vi "APC_9056_O2Control.vi"(1 "LoadIni?":bool, 2 "PC_ControlSettings":T1={"Spark advance [CADBTDC]"=0.0, "Pref"=0.0, "O2ref"=0.0, "DI advance [CADBTDC]"=0.0, "DI duration [ms] "=0.0, "CO2ref"=0.0, "PFI duration [ms]"=0.0, "IMEP ref"=0.0, "Speed ref"=0.0, "IGN enable"=TRUE, "DI enable"=TRUE, "CL PFI\n lambda"=TRUE, "CL PFI\nIMEP"=FALSE, "Activate\ncylinder"=[FALSE, FALSE, FALSE, FALSE, FALSE, FALSE], "Force idling"=FALSE, "Force motoring"=FALSE, "ETP resync"=FALSE, "Requested mode"=0, "Clear Sync Errors"=FALSE, "toggle TDC"=FALSE, "l ref"=0.0, "PID control references"={"NG"=FALSE, "Ar"=FALSE, "O2"=FALSE, "Intake vent"=FALSE, "Cross vent"=FALSE, "Exhaust vent"=FALSE, "NG control mode"=0, "NG-FC-001-REF"=0.0, "WF-OA-002-REF"=0.0, "IMEP-REF"=0.0, "Nm-REF"=0.0, "Ar control mode"=0, "AR-PC-002-REF"=0.0, "WF-PT-004-REF"=0.0, "O2 control mode"=0, "O2-FC-001-REF"=0.0, "WF-OA-001-REF"=0.0, "Tcoolant control  mode"=0, "EC-FC-001-REF"=0.0, "EC-TT-001-REF"=0.0, "Texh control mode"=0, "SW-FC-004-REF"=0.0, "SW-FT-002-REF"=0.0, "WF-TT-004-REF"=0.0, "Toil control mode"=0, "SW-FC-009-REF"=0.0, "SW-FT-004-REF"=0.0, "EO-TT-001-REF"=0.0, "AIC201_CO2_ConcTarget"=0.0, "O2_FF_NG"=FALSE, "Dyno control mode"=0, "Membrane control mode"=0, "AR-FT-001-REF"=0.0, "MTR modbus floats"=[0.0, 0.0, 0.0, 0.0, 0.0, 0.0, 0.0, 0.0, 0.0, 0.0, 0.0, 0.0, 0.0, 0.0, 0.0, 0.0, 0.0, 0.0, 0.0], "MTR modbus u16"=[0, 0, 0, 0, 0, 0, 0], "MTR HB"=FALSE, "PC_HB"=FALSE, "EMERGENCY STOP"=FALSE}, "CA50setpoint [CADATDC]"=0.0, "CA50 control"=TRUE, "Knock control"=TRUE, "CLEAR EMERGENCY STOP"=FALSE, "EMERGENCY STOP"=FALSE}, 3 "input cluster":T3) -> (0 "O2-FC-001-REF":dbl format="%.2f")   [LabVIEW 2020]
uses:
  controls/APC_PIDCluster.ctl
  controls/APC_ControlSettings.ctl
  controls/APC_PIDcontrolSettings.ctl
  controls/APC_cascadePIDsettings.ctl
  <vilib>/addons/control/pid/pid.llb/PID Advanced (DBL).vi
  <vilib>/Utility/xml.llb/Read From XML File(string).vi
  <vilib>/Utility/xml.llb/Write to XML File(string).vi
  <vilib>/addons/control/pid/NI_PID_pid.lvlib
panel:
  out "direct?":bool
  out "Direct control":dbl format="%.2f"
  in  "O2-FC-001-REF (manual)":dbl
  in  "O2/NG":dbl=3.0
  in  "compensate NG":bool
  in  "FT/FC?":bool
  in  "save":bool
  in  "load":bool
  out "O2 control mode":u8
  out "EC-TT-001":dbl
  in  "FF control":dbl format="%.2f"
  in  "reinitialize? (F)":bool
  in  "WF-OA-001-O2corr-REF (manual)":dbl
  in  "O2 control mode (manual)":u8
  in  "PID gains":T4={"proportional gain (Kc)"=1.0, "integral time (Ti, min)"=0.01, "derivative time (Td, min)"=0.0} {"derivative time (Td, min)" format="%.3f"; "integral time (Ti, min)" format="%.3f"; "proportional gain (Kc)" format="%.3f"}
  in  "PID setpoint range":cluster{"setpoint high":dbl, "setpoint low":dbl}={"setpoint high"=100.0, "setpoint low"=0.0} {"setpoint high" format="%.2f"; "setpoint low" format="%.2f"}
  in  "PID output range":cluster{"output high":dbl, "output low":dbl}={"output high"=100.0, "output low"=-100.0} {"output low" format="%.2f"; "output high" format="%.2f"}
  in  "Override PC PID references":bool
  in  "Safe mode control":dbl format="%.2f"
  in  "learn?":bool
  out "CL on?":bool
  out "setpoint":dbl format="%.2f"
  # "O2 control"
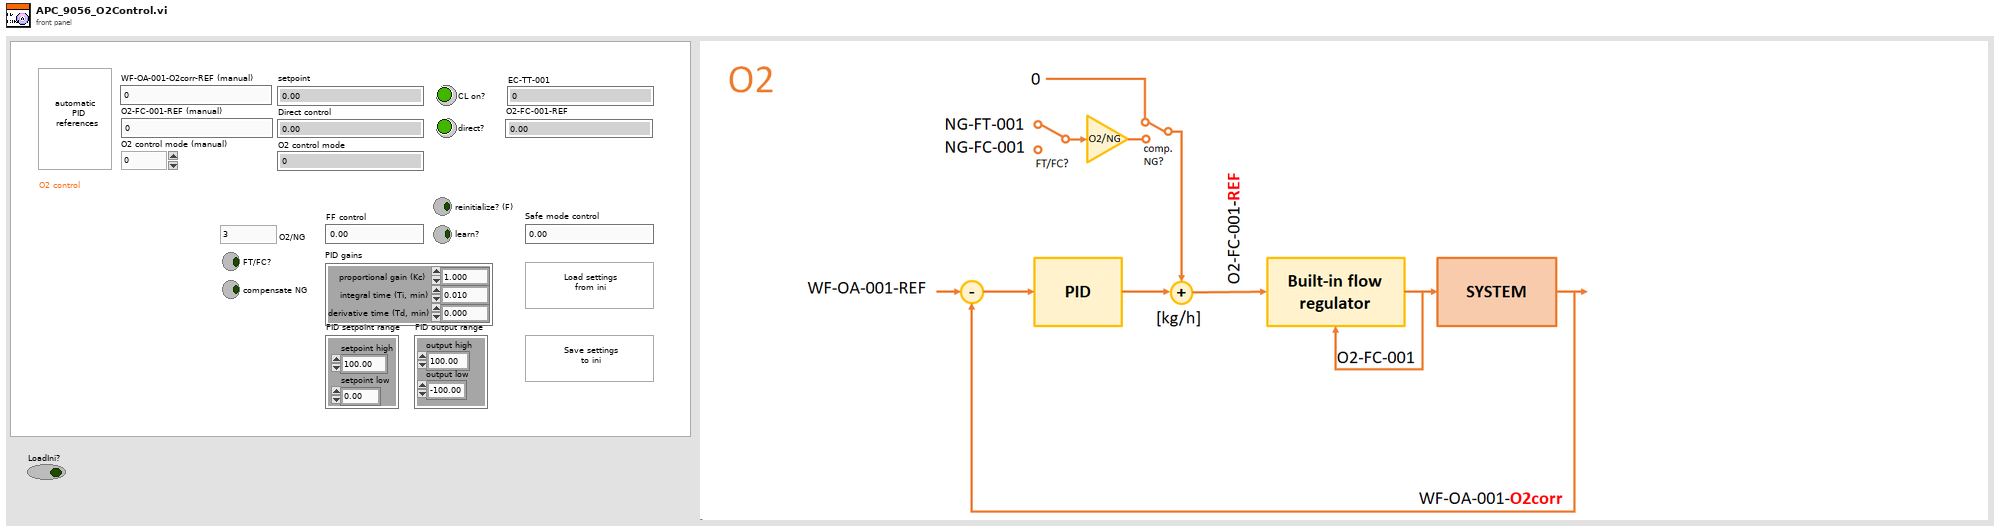
[diagram p1: front panel]
types:
  T1 = typedef "APC_ControlSettings.ctl" = cluster{"Spark advance [CADBTDC]":dbl, "Pref":dbl, "O2ref":dbl, "DI advance [CADBTDC]":dbl, "DI duration [ms] ":dbl, "CO2ref":dbl, "PFI duration [ms]":dbl, "IMEP ref":dbl, "Speed ref":dbl, "IGN enable":bool, "DI enable":bool, "CL PFI\n lambda":bool, "CL PFI\nIMEP":bool, "Activate\ncylinder":bool[], "Force idling":bool, "Force motoring":bool, "ETP resync":bool, "Requested mode":i8, "Clear Sync Errors":bool, "toggle TDC":bool, "l ref":dbl, "PID control references":T2, "CA50setpoint [CADATDC]":dbl, "CA50 control":bool, "Knock control":bool, "CLEAR EMERGENCY STOP":bool, "EMERGENCY STOP":bool}
  T2 = typedef "APC_PIDcontrolSettings.ctl" = cluster{"NG":bool, "Ar":bool, "O2":bool, "Intake vent":bool, "Cross vent":bool, "Exhaust vent":bool, "NG control mode":u8, "NG-FC-001-REF":dbl, "WF-OA-002-REF":dbl, "IMEP-REF":dbl, "Nm-REF":dbl, "Ar control mode":u8, "AR-PC-002-REF":dbl, "WF-PT-004-REF":dbl, "O2 control mode":u8, "O2-FC-001-REF":dbl, "WF-OA-001-REF":dbl, "Tcoolant control  mode":u8, "EC-FC-001-REF":dbl, "EC-TT-001-REF":dbl, "Texh control mode":u8, "SW-FC-004-REF":dbl, "SW-FT-002-REF":dbl, "WF-TT-004-REF":dbl, "Toil control mode":u8, "SW-FC-009-REF":dbl, "SW-FT-004-REF":dbl, "EO-TT-001-REF":dbl, "AIC201_CO2_ConcTarget":dbl, "O2_FF_NG":bool, "Dyno control mode":u8, "Membrane control mode":u8, "AR-FT-001-REF":dbl, "MTR modbus floats":sgl[], "MTR modbus u16":u16[], "MTR HB":bool, "PC_HB":bool, "EMERGENCY STOP":bool}
  T3 = typedef "APC_PIDCluster.ctl" = cluster{"AR-FT-001":dbl, "O2-FC-001":dbl, "SW-FT-004":dbl, "SW-FT-002":dbl, "WF-OA-002":dbl, "WF-PT-004":dbl, "WF-OA-001":dbl, "EC-TT-001":dbl, "WF-TT-004":dbl, "EC-FC-001":dbl, "NG-FC-001":dbl, "EO-TT-001":dbl, "SW-FC-008":dbl, "SW-FC-004":dbl, "IMEPn6":dbl, "TORQUE":dbl, "CylPresWarnings":dbl, "CylPresErrors":dbl, "NG-FT-001":dbl, "EngineSpeed_rpm":dbl}
  T4 = cluster{"proportional gain (Kc)":dbl, "integral time (Ti, min)":dbl, "derivative time (Td, min)":dbl}
  T5 = typedef "APC_cascadePIDsettings.ctl" = cluster{"HL FF control":dbl, "LL FF control":dbl, "HL PID gains":cluster{"proportional gain (Kc)":dbl, "integral time (Ti, min)":dbl, "derivative time (Td, min)":dbl}, "LL PID gains":cluster{"proportional gain (Kc)":dbl, "integral time (Ti, min)":dbl, "derivative time (Td, min)":dbl}, "HL PID setpoint range":cluster{"setpoint high":dbl, "setpoint low":dbl}, "HL PID output range":cluster{"output high":dbl, "output low":dbl}, "LL PID setpoint range":cluster{"setpoint high":dbl, "setpoint low":dbl}, "LL PID output range":cluster{"output high":dbl, "output low":dbl}, "Safe mode control":dbl}
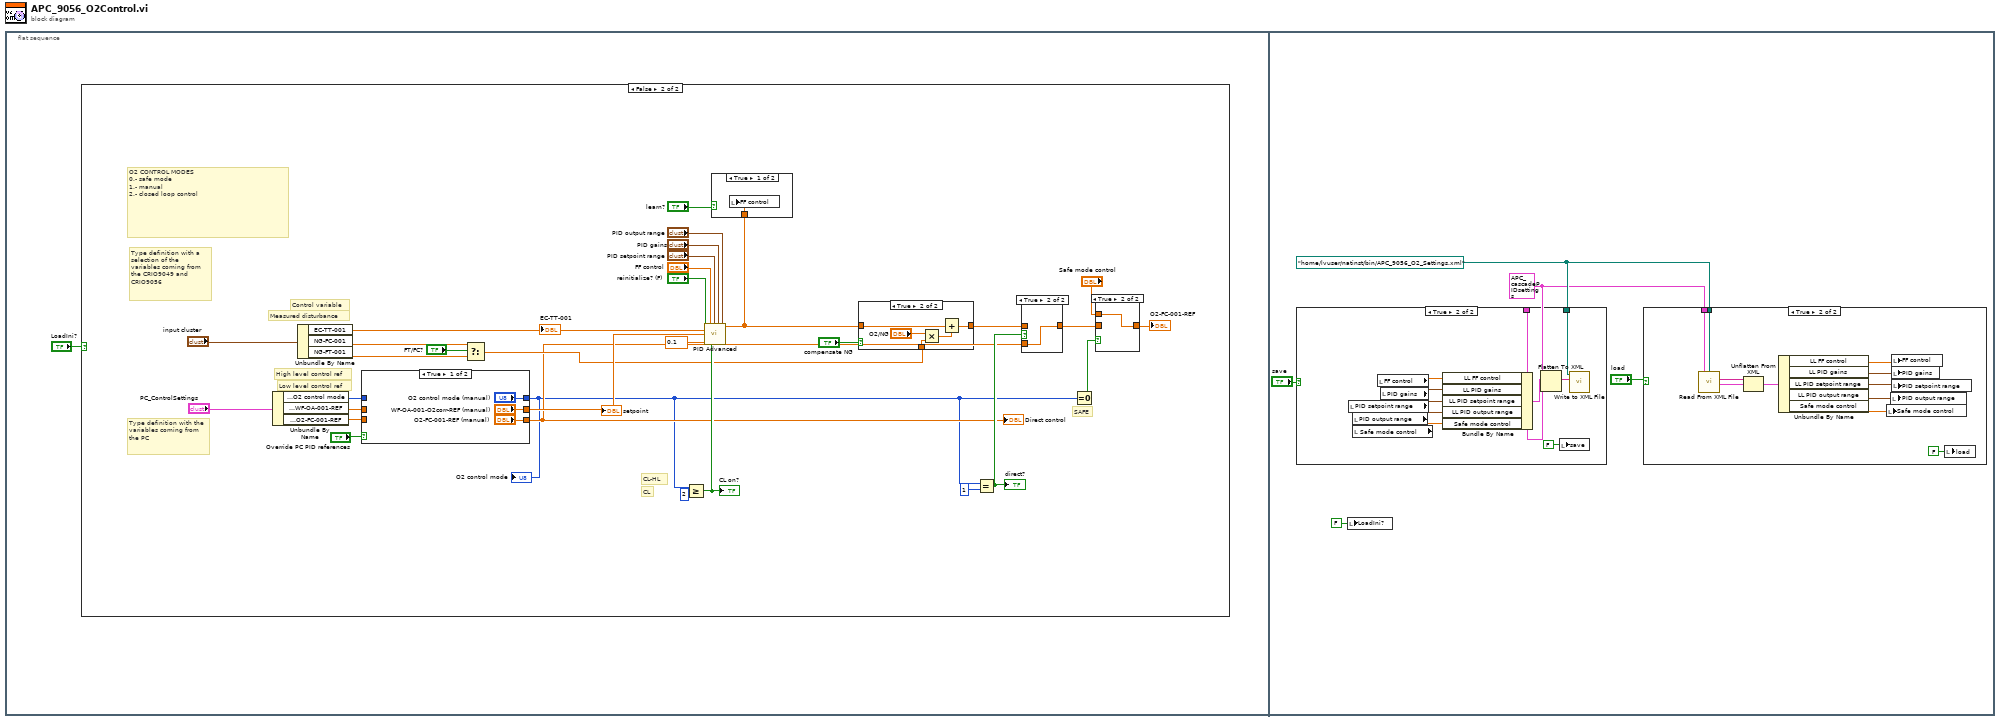
[diagram p0: block diagram]
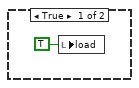
[diagram p2: hidden frame]
diagram:
  n1 = flat-sequence {
    frame #0 {
      n2 = case shown="False" "LoadIni?" {
        frame True {
          n3 = local write "load"(TRUE ("load")) -> ()
        }
        frame False {
          # "Type definition with a selection of the variables coming from the CRIO9049 and CRIO9056"
          # "Type definition with the variables coming from the PC"
          # "Low level control ref"
          # "Measured disturbance"
          # "High level control ref"
          # "Control variable"
          # "SAFE"
          # "CL-HL"
          # "CL"
          # "O2 CONTROL MODES\n0.- safe mode\n1.- manual\n2.- closed loop control"
          n4 = Unbundle By Name("PC_ControlSettings") -> ("PID control references.O2 control mode"=w22:u8, "PID control references.WF-OA-001-REF"=w21:dbl, "PID control references.O2-FC-001-REF"=w9:dbl)
          n5 = Unbundle By Name("input cluster") -> ("EC-TT-001"=w19:dbl, "NG-FC-001"=w15:dbl, "NG-FT-001"=w14:dbl)
          "EC-TT-001" <- w19
          n6 = case shown="True" "Override PC PID references" {
            tunnel: w22 -> [_ w51]
            tunnel: w21 -> [_ w50]
            tunnel: ["O2 control mode (manual)" w51] -> w3
            tunnel: ["WF-OA-001-O2corr-REF (manual)" w50] -> w16
            tunnel: w9 -> [_ w49]
            tunnel: ["O2-FC-001-REF (manual)" w49] -> w4
            frame True {
            }
            frame False {
            }
          }
          "setpoint" <- w16
          "O2 control mode" <- w3
          "Direct control" <- w4
          n7 = Select(t=w15, s="FT/FC?", f=w14) -> (s? t:f=w10:dbl)
          n8 = Greater Or Equal?(x=w3, y=u8 2) -> (x >= y?=w32:bool)
          "CL on?" <- w32
          n9 = call-poly <vilib>:"PID Advanced.vi"("setpoint"=w16, "output range"="PID output range", "auto? (T)"=w32, "manual control"="FF control", "process variable"=w19, "setpoint range"="PID setpoint range", "PID gains"="PID gains", "dt (s)"=0.1, "reinitialize? (F)"="reinitialize? (F)") -> ("output"=w11:dbl)  [unwired: 5 in, 1 out]
          n10 = case shown="True" "learn?" {
            tunnel: w11 -> [w43 _]
            frame True {
              n11 = local write "FF control"(w43) -> ()
            }
            frame False {
            }
          }
          n12 = case shown="True" "compensate NG" {
            tunnel: w11 -> [w37 w41]
            tunnel: [w37 w42] -> w5
            tunnel: w10 -> [_ w39]
            frame False {
            }
            frame True {
              n13 = Multiply(x="O2/NG", y=w39) -> (x*y=w40:dbl)
              n14 = Add(x=w41, y=w40) -> (x+y=w42:dbl)
            }
          }
          n15 = Equal?(x=w3, y=u8 1) -> (x = y?=w7:bool)
          "direct?" <- w7
          n16 = case shown="True" w7 {
            tunnel: [w35 w36] -> w6
            tunnel: w5 -> [w35 _]
            tunnel: w4 -> [_ w36]
            frame False {
            }
            frame True {
            }
          }
          n17 = Equal To 0?(x=w3) -> (x = 0?=w34:bool)
          n18 = case shown="True" w34 {
            tunnel: [w44 w45] -> w28
            tunnel: "Safe mode control" -> [_ w45]
            tunnel: w6 -> [w44 _]
            frame False {
            }
            frame True {
            }
          }
          "O2-FC-001-REF" <- w28
        }
      }
    }
    frame #1 {
      w54 = path "/home/lvuser/natinst/bin/APC_9056_O2_Settings.xml" ("XML File Path")
      w53 = T5 {"HL FF control"=0.0, "LL FF control"=0.0, "HL PID gains"={"proportional gain (Kc)"=1.0, "integral time (Ti, min)"=0.01, "derivative time (Td, min)"=0.0}, "LL PID gains"={"proportional gain (Kc)"=1.0, "integral time (Ti, min)"=0.01, "derivative time (Td, min)"=0.0}, "HL PID setpoint range"={"setpoint high"=100.0, "setpoint low"=0.0}, "HL PID output range"={"output high"=0.0, "output low"=0.0}, "LL PID setpoint range"={"setpoint high"=100.0, "setpoint low"=0.0}, "LL PID output range"={"output high"=10.0, "output low"=-10.0}, "Safe mode control"=0.0} ("Cluster")
      n19 = case shown="True" "save" {
        tunnel: w54 -> [_ w69]
        tunnel: w53 -> [_ w68]
        frame False {
        }
        frame True {
          n20 = local read "PID setpoint range"() -> (w74:cluster{"setpoint high":dbl, "setpoint low":dbl})
          n21 = local read "PID output range"() -> (w73:cluster{"output high":dbl, "output low":dbl})
          n22 = local read "Safe mode control"() -> (w72:dbl)
          n23 = local read "FF control"() -> (w76:dbl)
          n24 = local read "PID gains"() -> (w75:T4)
          n25 = Bundle By Name(cluster=w68, "LL FF control"=w76, "LL PID gains"=w75, "LL PID setpoint range"=w74, "LL PID output range"=w73, "Safe mode control"=w72) -> (w71:T5)
          n26 = Flatten To XML(6:w71) -> (2:w70:string)
          n27 = local write "save"(FALSE ("load")) -> ()
          n28 = call-poly <vilib>:"Write to XML File.vi"("XML Input"=w70, "XML File Path"=w69) -> ()  [unwired: 7 in, 3 out]
        }
      }
      n29 = local write "LoadIni?"(FALSE ("LoadIni?")) -> ()
      n30 = case shown="True" "load" {
        tunnel: w54 -> [_ w65]
        tunnel: w53 -> [_ w64]
        frame False {
        }
        frame True {
          n31 = call-poly <vilib>:"Read From XML File.vi"("XML File Path"=w65) -> ("XML Elements"=w66:string)  [unwired: 8 in, 2 out]
          n32 = Unflatten From XML(xml string=w66, type=w64) -> (value=w63:T5)  [unwired: 1 in, 1 out]
          n33 = Unbundle By Name(w63) -> ("LL FF control"=w62:dbl, "LL PID gains"=w61:T4, "LL PID setpoint range"=w60:cluster{"setpoint high":dbl, "setpoint low":dbl}, "LL PID output range"=w59:cluster{"output high":dbl, "output low":dbl}, "Safe mode control"=w58:dbl)
          n34 = local write "Safe mode control"(w58) -> ()
          n35 = local write "PID output range"(w59) -> ()
          n36 = local write "FF control"(w62) -> ()
          n37 = local write "PID gains"(w61) -> ()
          n38 = local write "PID setpoint range"(w60) -> ()
          n39 = local write "load"(FALSE ("save")) -> ()
        }
      }
    }
  }
